vi "Sync.Acquire.vi"(8 "error in (no error)":errorcluster, 11 "DAQmx in":refnum<class "DAQmx.lvclass">) -> (0 "error out":errorcluster, 3 "DAQmx out":refnum<class "DAQmx.lvclass">)   [LabVIEW 2019, in "DAQmx.lvclass"]
uses:
  DAQmx.lvclass
  DAQmx.lvclass/DAQmx.ctl
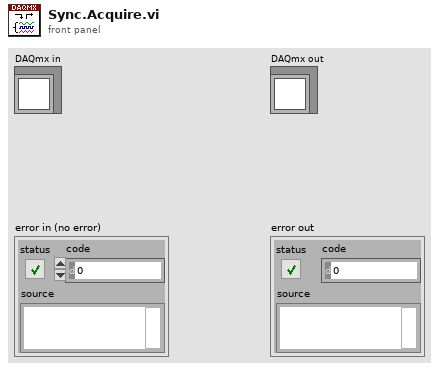
[diagram p1: front panel]
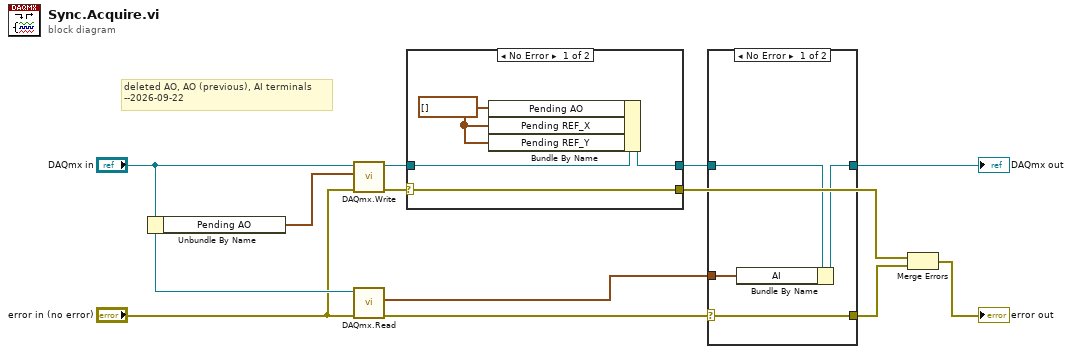
[diagram p0: block diagram]
diagram:
  # "deleted AO, AO (previous), AI terminals\n--2026-09-22"
  n1 = Unbundle By Name("DAQmx in") -> ("Pending AO"=w7:waveform(dbl)[])
  n2 = call "DAQmx.Write.vi"("error in (no error)"="error in (no error)", "AOwfm"=w7, "DAQmx in"="DAQmx in") -> ("error out"=w12:errorcluster, "DAQmx out"=w11:refnum<class "DAQmx.lvclass">)  [unwired: 6 in, 1 out]
  n3 = call "DAQmx.Read.vi"("error in"="error in (no error)", "DAQmx in"="DAQmx in") -> ("error out"=w6:errorcluster, "AIwfm"=w10:waveform(dbl)[])  [unwired: 6 in, 2 out]
  n4 = case shown="No Error" w12 {
    selector: w12 -> [w16 w18]
    tunnel: [w16 w18] -> w5
    tunnel: w11 -> [w15 w17]
    tunnel: [w14 w17] -> w9
    frame No Error {
      w13 = waveform(dbl)[] [] ("Recovery.Pending AO")
      n5 = Bundle By Name(cluster=w15, "Pending AO"=w13, "Pending REF_X"=w13, "Pending REF_Y"=w13) -> (w14:refnum<class "DAQmx.lvclass">)
    }
    frame Error {
    }
  }
  n6 = case shown="No Error" w6 {
    selector: w6 -> [w19 w23]
    tunnel: w10 -> [w22 _]
    tunnel: w9 -> [w21 w24]
    tunnel: [w20 w24] -> w8
    tunnel: [w19 w23] -> w4
    frame No Error {
      n7 = Bundle By Name(cluster=w21, "AI"=w22) -> (w20:refnum<class "DAQmx.lvclass">)
    }
    frame Error {
    }
  }
  "DAQmx out" <- w8
  n8 = Merge Errors(w5, w4) -> (→"error out":errorcluster)
